vi "Set Temperature.vi"(8 "error in (no error)":errorcluster, 10 "Setpoint":dbl, 11 "Huber Settings":T1) -> (0 "error out":errorcluster, 1 "Connection Error":bool, 3 "Huber Settings":T1)   [LabVIEW 2018, in "Huber Ministat 230 TCU.lvlib"]
uses:
  Huber Ministat 230 TCU.lvlib
  Huber Settings.ctl
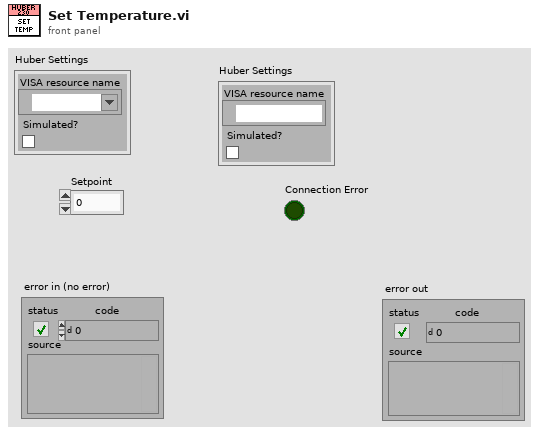
[diagram p1: front panel]
types:
  T1 = typedef "Huber Ministat 230 TCU.lvlib/Huber Settings.ctl" = cluster{"VISA resource name":refnum<visa-resource-name>, "Simulated?":bool}
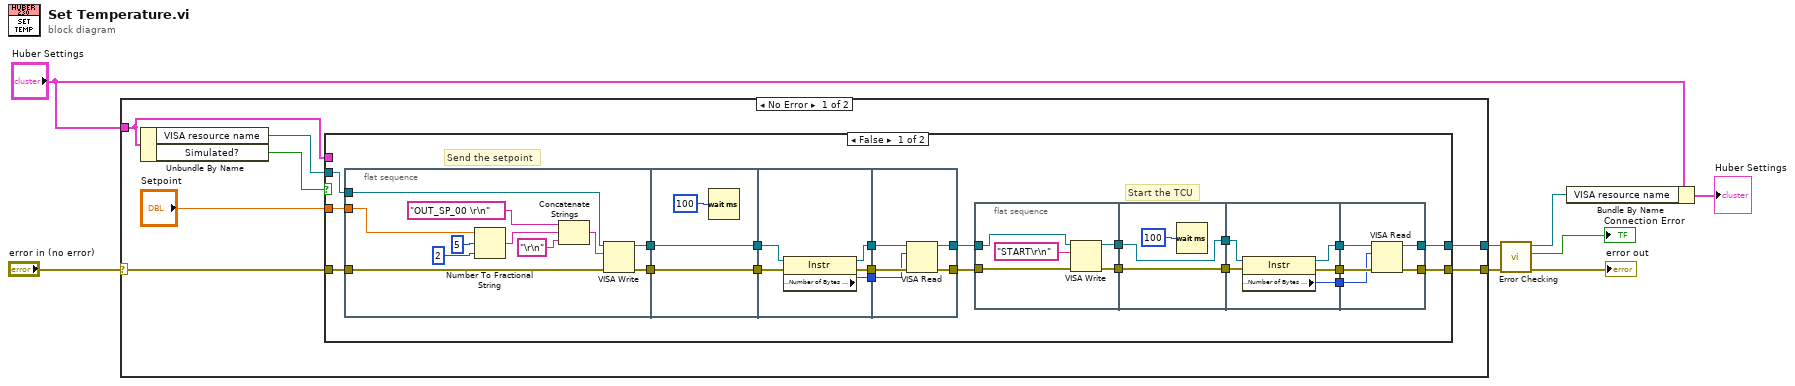
[diagram p0: block diagram]
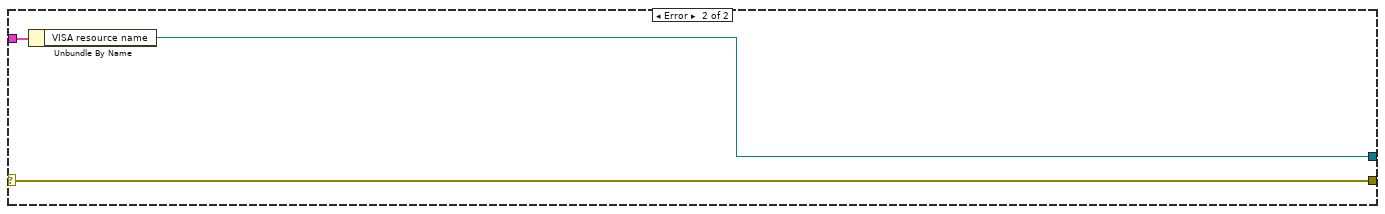
[diagram p3: hidden frame]
diagram:
  n1 = case shown="No Error" "error in (no error)" {
    selector: "error in (no error)" -> [w15 w83]
    tunnel: "Huber Settings" -> [w10 w82]
    tunnel: [w14 w83] -> w6
    tunnel: [w12 w81] -> w7
    frame No Error {
      n2 = Unbundle By Name(w10) -> ("VISA resource name"=w13:refnum<visa-resource-name>, "Simulated?"=w11:bool)
      n3 = case shown="False" w11 {
        tunnel: w15 -> [w35 w80]
        tunnel: [w17 w80] -> w14
        tunnel: [w18 w79] -> w12
        tunnel: w13 -> [w36 w79]
        tunnel: w10 -> [_ _]
        tunnel: "Setpoint" -> [w16 _]
        frame False {
          # "Start the TCU"
          # "Send the setpoint"
          n4 = flat-sequence {
            tunnel: [w65] -> w34
            tunnel: [w64] -> w33
            tunnel: w36 -> [w63]
            tunnel: w35 -> [w62]
            tunnel: w16 -> [w58]
            tunnel: w34 -> [w67]
            tunnel: w33 -> [w66]
            tunnel: [w67] -> w32
            tunnel: [w66] -> w31
            tunnel: [w71] -> w30
            tunnel: [w70] -> w29
            tunnel: [w69] -> w28
            tunnel: w32 -> [w73]
            tunnel: w31 -> [w72]
            tunnel: [w78] -> w19
            tunnel: [w77] -> w20
            tunnel: w30 -> [w76]
            tunnel: w29 -> [w75]
            tunnel: w28 -> [w74]
            frame #0 {
              n5 = Number To Fractional String(number=w58, width (-)=i16 5, precision (6)=i16 2) -> (F-format string=w61:string)  [unwired: 1 in]
              n6 = Concatenate Strings("OUT_SP_00 \r\n" ("string"), w61, "\r\n" ("string")) -> (w55:string)
              n7 = VISA Write(VISA resource name=w63, write buffer=w55, error in (no error)=w62) -> (VISA resource name out=w65:refnum<visa-resource-name>, error out=w64:errorcluster)  [unwired: 1 out]
            }
            frame #1 {
              n8 = Wait (ms)(milliseconds to wait=u32 100) -> ()  [unwired: 1 out]
            }
            frame #2 {
              n9 = property class="Instr"(reference=w73, error in=w72) -> (reference out=w71:refnum<visa-resource-name>, error out=w70:errorcluster, "Serial Settings:Number of Bytes at Serial Port"=w69:u32)
            }
            frame #3 {
              n10 = VISA Read(VISA resource name=w76, byte count=w74, error in (no error)=w75) -> (VISA resource name out=w77:refnum<visa-resource-name>, error out=w78:errorcluster)  [unwired: 2 out]
            }
          }
          n11 = flat-sequence {
            tunnel: [w41] -> w27
            tunnel: [w40] -> w26
            tunnel: w20 -> [w39]
            tunnel: w19 -> [w38]
            tunnel: w27 -> [w43]
            tunnel: w26 -> [w42]
            tunnel: [w43] -> w25
            tunnel: [w42] -> w24
            tunnel: [w47] -> w23
            tunnel: [w46] -> w22
            tunnel: [w45] -> w21
            tunnel: w25 -> [w49]
            tunnel: w24 -> [w48]
            tunnel: [w54] -> w17
            tunnel: [w53] -> w18
            tunnel: w23 -> [w52]
            tunnel: w22 -> [w51]
            tunnel: w21 -> [w50]
            frame #0 {
              n12 = VISA Write(VISA resource name=w39, write buffer="START\r\n", error in (no error)=w38) -> (VISA resource name out=w41:refnum<visa-resource-name>, error out=w40:errorcluster)  [unwired: 1 out]
            }
            frame #1 {
              n13 = Wait (ms)(milliseconds to wait=u32 100) -> ()  [unwired: 1 out]
            }
            frame #2 {
              n14 = property class="Instr"(reference=w49, error in=w48) -> (reference out=w47:refnum<visa-resource-name>, error out=w46:errorcluster, "Serial Settings:Number of Bytes at Serial Port"=w45:u32)
            }
            frame #3 {
              n15 = VISA Read(VISA resource name=w52, byte count=w50, error in (no error)=w51) -> (VISA resource name out=w53:refnum<visa-resource-name>, error out=w54:errorcluster)  [unwired: 2 out]
            }
          }
        }
        frame True {
        }
      }
    }
    frame Error {
      n16 = Unbundle By Name(w82) -> ("VISA resource name"=w81:refnum<visa-resource-name>)
    }
  }
  n17 = call "Error Checking.vi"("error in (no error)"=w6, "VISA resource name"=w7) -> ("error out"=→"error out":errorcluster, "Connection Error"=→"Connection Error":bool, "VISA resource name"=w4:refnum<visa-resource-name>)  [unwired: 7 in]
  n18 = Bundle By Name(cluster="Huber Settings", "VISA resource name"=w4) -> (→"Huber Settings":T1)
